vi "Stepping.vi"(6 "Microstep size":T1(ring), 7 "Speed":u32=5, 8 "error in (no error)":errorcluster, 9 "Direction":bool, 10 "Stepper motor":enum16{"X-axis", "Y-axis"}(ring), 11 "Steps":i32) -> (0 "error out":errorcluster)   [LabVIEW 2017]
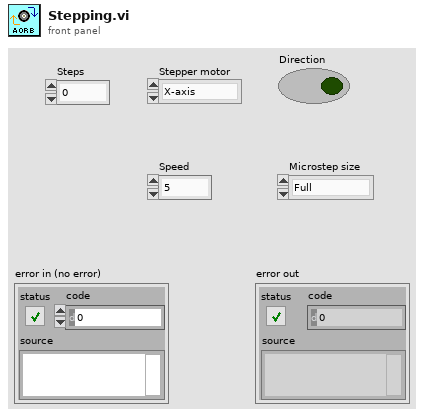
[diagram p1: front panel]
types:
  T1 = enum16{"Full", "Half", "Quarter", "Eighth", "Sixteenth"}
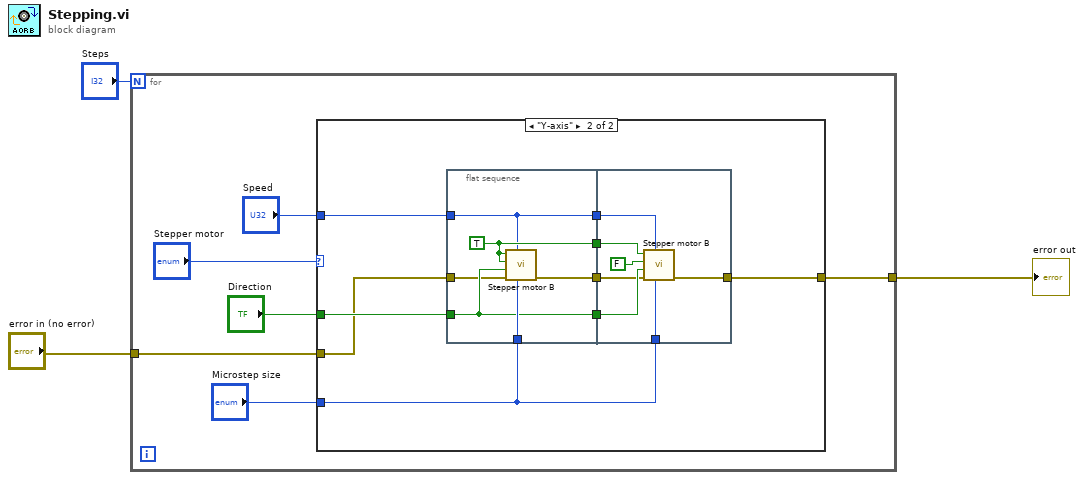
[diagram p0: block diagram]
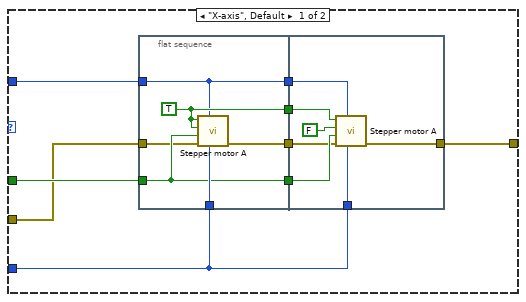
[diagram p2: hidden frame]
diagram:
  n1 = for {
    N: "Steps" -> [_]
    tunnel: "error in (no error)" -> [w6]
    tunnel: [w5] -> w1
    n2 = case shown="\"Y-axis\"" "Stepper motor" {
      tunnel: "Microstep size" -> [w15 w37]
      tunnel: "Direction" -> [w16 w38]
      tunnel: "Speed" -> [w14 w36]
      tunnel: w6 -> [w11 w32]
      tunnel: [w10 w33] -> w5
      frame "X-axis", Default {
        n3 = flat-sequence {
          tunnel: [w24] -> w18
          tunnel: [w22] -> w17
          tunnel: w15 -> [w23]
          tunnel: w16 -> [w22]
          tunnel: w14 -> [w21]
          tunnel: [w21] -> w13
          tunnel: [w20] -> w12
          tunnel: w11 -> [w19]
          tunnel: w18 -> [w31]
          tunnel: w17 -> [w29]
          tunnel: w15 -> [w28]
          tunnel: w13 -> [w27]
          tunnel: w12 -> [w26]
          tunnel: [w25] -> w10
          frame #0 {
            w24 = TRUE
            n4 = call "Stepper motor A.vi"("Microstep size"=w23, "Speed"=w21, "error in (no error)"=w19, "Direction (C/DIO4 (DIO4))"=w22, "Step (C/DIO3 (DIO3))"=w24, "Enable (C/DIO2 (DIO2))"=w24) -> ("error out"=w20:errorcluster)  [unwired: 5 in]
          }
          frame #1 {
            n5 = call "Stepper motor A.vi"("Microstep size"=w28, "Speed"=w27, "error in (no error)"=w26, "Direction (C/DIO4 (DIO4))"=w29, "Step (C/DIO3 (DIO3))"=FALSE, "Enable (C/DIO2 (DIO2))"=w31) -> ("error out"=w25:errorcluster)  [unwired: 5 in]
          }
        }
      }
      frame "Y-axis" {
        n6 = flat-sequence {
          tunnel: [w46] -> w40
          tunnel: [w44] -> w39
          tunnel: w37 -> [w45]
          tunnel: w38 -> [w44]
          tunnel: w36 -> [w43]
          tunnel: [w43] -> w35
          tunnel: [w42] -> w34
          tunnel: w32 -> [w41]
          tunnel: w40 -> [w53]
          tunnel: w39 -> [w51]
          tunnel: w37 -> [w50]
          tunnel: w35 -> [w49]
          tunnel: w34 -> [w48]
          tunnel: [w47] -> w33
          frame #0 {
            w46 = TRUE
            n7 = call "Stepper motor B.vi"("Microstep size"=w45, "Speed"=w43, "error in (no error)"=w41, "Direction (A/DIO5 (Pin 21))"=w44, "Step (A/DIO4 (Pin 19))"=w46, "Enable (A/DIO0 (Pin 11))"=w46) -> ("error out"=w42:errorcluster)  [unwired: 4 in, 1 out]
          }
          frame #1 {
            n8 = call "Stepper motor B.vi"("Microstep size"=w50, "Speed"=w49, "error in (no error)"=w48, "Direction (A/DIO5 (Pin 21))"=w51, "Step (A/DIO4 (Pin 19))"=FALSE, "Enable (A/DIO0 (Pin 11))"=w53) -> ("error out"=w47:errorcluster)  [unwired: 4 in, 1 out]
          }
        }
      }
    }
  }
  "error out" <- w1
